vi "Training_model.vi"() -> ()   [LabVIEW 2018]
uses:
  <vilib>/Utility/file.llb/Read Delimited Spreadsheet (DBL).vi
  <vilib>/Utility/file.llb/Write Delimited Spreadsheet (DBL).vi
panel:
  in  "Tab Control":enum32{"Training model", "Debugging stuff"}(tab)
  out "Y data":dbl[][](graph)
  in  "Model Selector":enum16{"Standard_MLP", "Deep_MLP", "Light_MLP"}(ring)
  out "X data":dbl[][](graph)
  in  "stop":bool
  in  "Training Button":bool
  out "Model Path":string
  out "Python error":string
  out "all rows":dbl[][](array[numeric])
  out "String":string="\"C:\\\\Users\\genyd\\AppData\\Local\\Microsoft\\WindowsApps\\python3.12.exe\" \"C:\\Users\\genyd\\OneDrive\\Documentos\\Trabajos\\Personales\\SURE\\ZEUS\\Training data\\LabVIEW_training.py\""
  out "standard output":string
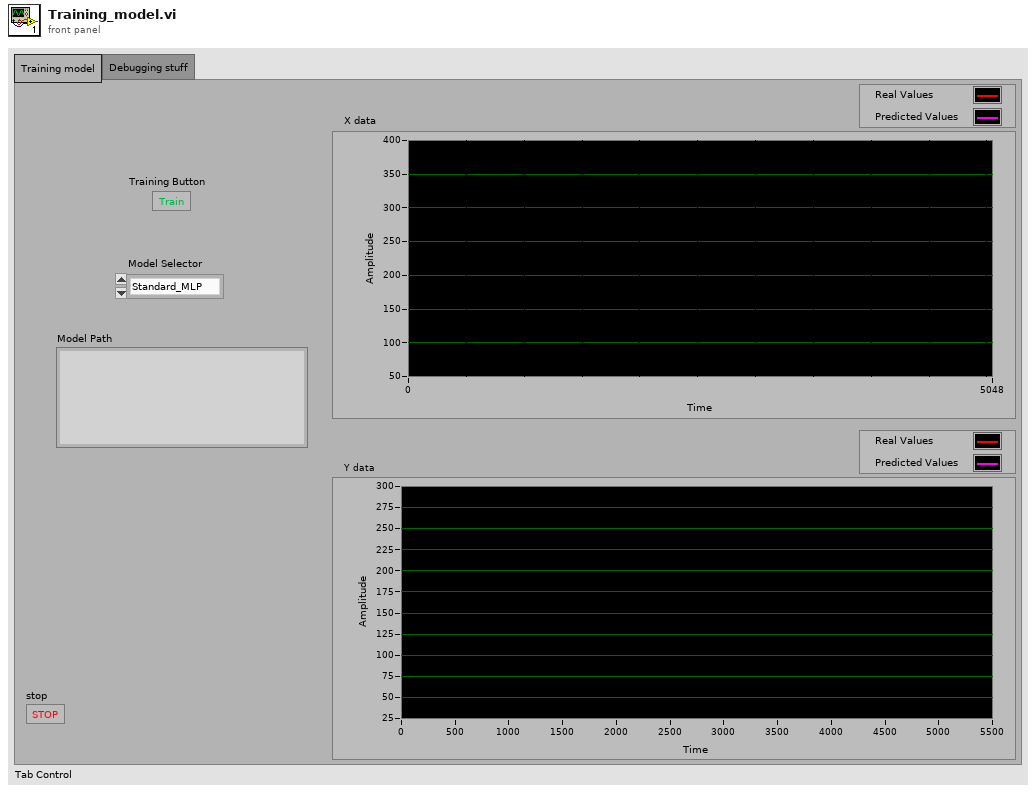
[diagram p1: front panel]
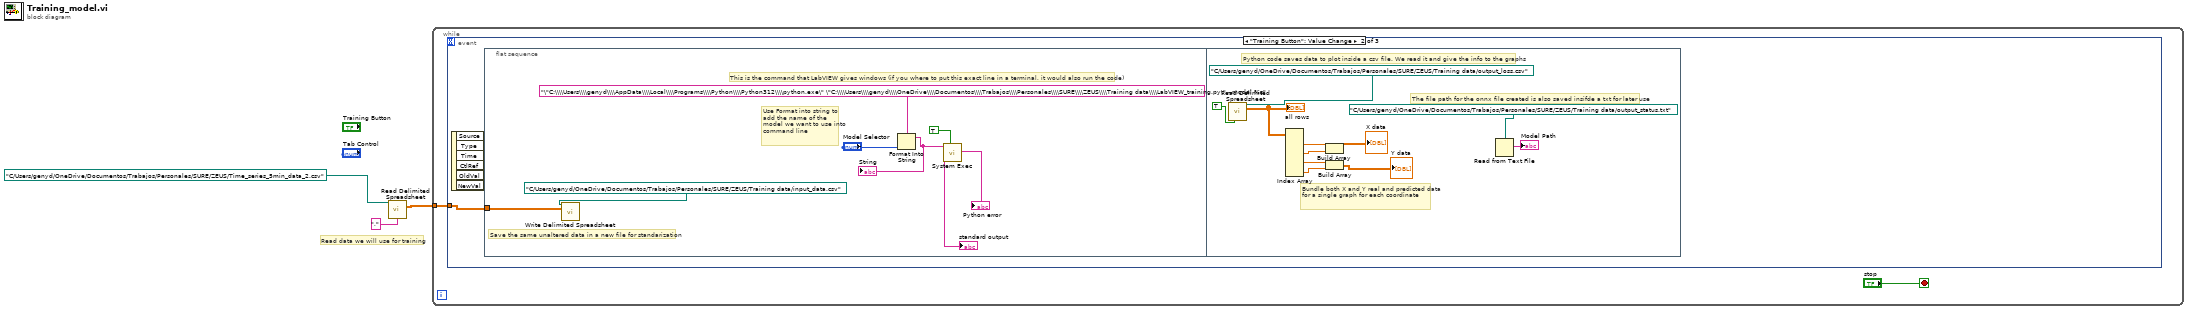
[diagram p0: block diagram]
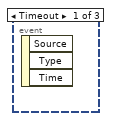
[diagram p2: hidden frame]
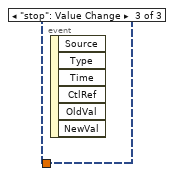
[diagram p3: hidden frame]
diagram:
  # "Read data we will use for training"
  n1 = call-poly <vilib>:"Read Delimited Spreadsheet.vi"("file path (dialog if empty)"=path "C:/Users/genyd/OneDrive/Documentos/Trabajos/Personales/SURE/ZEUS/Time_series_5min_data_2.csv", "delimiter (\\t)"="," ("delimiter (\\t)")) -> ("all rows"=w1:dbl[][])  [unwired: 8 in, 5 out]
  n2 = while {
    tunnel: w1 -> [w4]
    stop <- "stop" stop-if-true
    n3 = event shown="[1] \"Training Button\": Value Change" {
      selector: _ -> [_ _ _]
      dyn-events: _ -> [_ _ _]
      timeout: _ -> [_ _ _]
      tunnel: w4 -> [_ w6 _]
      event Timeout {
        n4 = event-data() -> ()  [unwired: 1 in, 3 out]
      }
      event "Training Button": Value Change {
        n5 = event-data() -> ()  [unwired: 1 in, 6 out]
        n6 = flat-sequence {
          tunnel: w6 -> [w14]
          frame #0 {
            # "Use Format into string to add the name of the model we want to use into command line"
            # "This is the command that LabVIEW gives windows (if you where to put this exact line in a terminal, it would also run the code)"
            # "Save the same unaltered data in a new file for standarization"
            n7 = call-poly <vilib>:"Write Delimited Spreadsheet.vi"("file path (dialog if empty)"=path "C:/Users/genyd/OneDrive/Documentos/Trabajos/Personales/SURE/ZEUS/Training data/input_data.csv" ("new file path (Not A Path if cancelled)"), "2D data"=w14) -> ()  [unwired: 12 in, 2 out]
            n8 = Format Into String(format string="\"C:\\\\Users\\\\genyd\\\\AppData\\\\Local\\\\Programs\\\\Python\\\\Python312\\\\python.exe\" \"C:\\\\Users\\\\genyd\\\\OneDrive\\\\Documentos\\\\Trabajos\\\\Personales\\\\SURE\\\\ZEUS\\\\Training data\\\\LabVIEW_training.py\" --model %s", "Model Selector") -> (resulting string=w8:string)  [unwired: 2 in, 1 out]
            "String" <- w8
            n9 = call <vilib>:"System Exec.vi"("wait until completion? (T)"=TRUE, "command line"=w8) -> ("standard error"=→"Python error":string, "standard output"=→"standard output":string)  [unwired: 6 in, 2 out]
          }
          frame #1 {
            # "Bundle both X and Y real and predicted data for a single graph for each coordinate"
            # "The file path for the onnx file created is also saved insifde a txt for later use"
            # "Python code saves data to plot inside a csv file. We read it and give the info to the graphs"
            n10 = call-poly <vilib>:"Read Delimited Spreadsheet.vi"("file path (dialog if empty)"=path "C:/Users/genyd/OneDrive/Documentos/Trabajos/Personales/SURE/ZEUS/Training data/output_loss.csv", "transpose? (F)"=TRUE) -> ("all rows"=w19:dbl[][])  [unwired: 8 in, 5 out]
            "all rows" <- w19
            n11 = Index Array(array=w19) -> (element #1=w20:dbl[], element #2=w21:dbl[], element #3=w23:dbl[], element #4=w24:dbl[])  [unwired: 8 in]
            n12 = Build Array(w20, w21) -> (→"X data":dbl[][])
            n13 = Build Array(w23, w24) -> (→"Y data":dbl[][])
            n14 = Read from Text File(file (use dialog)=path "C:/Users/genyd/OneDrive/Documentos/Trabajos/Personales/SURE/ZEUS/Training data/output_status.txt") -> (text=→"Model Path":string)  [unwired: 3 in, 3 out]
          }
        }
      }
      event "stop": Value Change {
        n15 = event-data() -> ()  [unwired: 1 in, 6 out]
      }
    }
  }
